vi "Begin.vi"() -> (0 "error out":errorcluster)   [LabVIEW 2013]
doc: "Called before other user functions, this VI is expected to open initial I/O refnums, load in file data, and do all program initialization. Notice that the <B>error out</B> terminal is simply used for data flow. Wiring it to other structures or subVIs ensures that this VI runs first."
uses:
  <vilib>/Rock Robotics/SystemInterfaces/DIO/FPGA_DIOPWMChannel.ctl
  <vilib>/Rock Robotics/WPI/DriverStation/WPI_DriverStationRobotMode2.ctl
  <vilib>/Rock Robotics/WPI/Joystick/WPI_JoystickDeviceEnum.ctl
  <vilib>/Rock Robotics/SystemInterfaces/DIO/FPGA_DIOChannel.ctl
  <vilib>/Rock Robotics/WPI/SafetyOutput/WPI_SafetyOutputConfigMenu.ctl
  <vilib>/Rock Robotics/SystemInterfaces/Typedef/FPGA_TypedefAnalogModule.ctl
  <vilib>/Rock Robotics/SystemInterfaces/AI/FPGA_AIChannel.ctl
  <vilib>/Rock Robotics/SystemInterfaces/Typedef/FPGA_TypedefAnalogModuleForGyro.ctl
  <vilib>/Rock Robotics/SystemInterfaces/AI/FPGA_AIGyroChannel.ctl
  <vilib>/Rock Robotics/SystemInterfaces/Typedef/FPGA_TypedefDigitalModule.ctl
  Robot Global Data.vi
  <vilib>/Rock Robotics/WPI/MotorControl/WPI_MotorControlOpen Jaguar.vi
  <vilib>/Rock Robotics/WPI/RobotDrive/WPI_RobotDriveOpen4MotorWithJaguar.vi
  <vilib>/Rock Robotics/WPI/MotorControl/WPI_MotorControlOpen Talon.vi
panel:
  out "error out 2":errorcluster
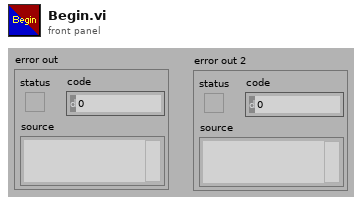
[diagram p1: front panel]
types:
  T1 = typedef "FPGA_DIOChannel.ctl" = enum8{"DIO 1", "DIO 2", "DIO 3", "DIO 4", "DIO 5", "DIO 6", "DIO 7", "DIO 8", "DIO 9", "DIO 10", "DIO 11", "DIO 12", "DIO 13", "DIO 14", "Invalid"}
  T2 = typedef "FPGA_TypedefDigitalModule.ctl" = enum16{"Digital Module 1", "Digital Module 2"}
  T3 = typedef "FPGA_AIGyroChannel.ctl" = enum8{"AI 1", "AI 2", "Invalid"}
  T4 = typedef "FPGA_TypedefAnalogModuleForGyro.ctl" = enum16{"Analog Module 1"}
  T5 = typedef "FPGA_AIChannel.ctl" = enum8{"AI 1", "AI 2", "AI 3", "AI 4", "AI 5", "AI 6", "AI 7", "AI 8", "Invalid"}
  T6 = typedef "FPGA_TypedefAnalogModule.ctl" = enum16{"Analog Module 1", "Analog Module 2"}
  T7 = typedef "WPI_SafetyOutputConfigMenu.ctl" = enum16{"Enable", "Disable"}
  T8 = typedef "FPGA_DIOPWMChannel.ctl" = enum8{"PWM 1", "PWM 2", "PWM 3", "PWM 4", "PWM 5", "PWM 6", "PWM 7", "PWM 8", "PWM 9", "PWM 10", "Invalid"}
  T9 = typedef "WPI_JoystickDeviceEnum.ctl" = enum16{"USB 1", "USB 2", "USB 3", "USB 4", "Kinect 1", "Kinect 2"}
  T10 = typedef "WPI_DriverStationRobotMode2.ctl" = enum16{"Autonomous Disabled", "Autonomous Enabled", "Teleop Disabled", "Teleop Enabled", "Timeout", "Finish", "Test Disabled", "Test Enabled"}
  T11 = typedef "WPI_GyroDevRef.ctl" = cluster{"DevStatus":errorcluster, "Analog Module":T6, "Analog Channel":T5, "Offset":dbl, "Gain (VoltsPerDegree/Second)":dbl}
  T12 = typedef "WPI_AnalogChannelDevRef.ctl" = cluster{"DevStatus":errorcluster, "Analog Module":T6, "Analog Channel":T5}
  T13 = typedef "WPI_RobotDriveDevRef.ctl" = cluster{"DevStatus":errorcluster, "Motors[]":T14[], "Square Inputs":bool, "Max Output":dbl, "Isochronous":bool}
  T14 = typedef "WPI_MotorControlDeviceRef.ctl" = cluster{"DeviceStatus":errorcluster, "Type":enum16{"PWM", "CAN"}, "PWM":cluster{"Digital Module":T2, "PWM Channel":T8, "DeadBand":T15}, "CAN":cluster{"Device Number":u8, "Control Mode":T16, "Semaphore":T17, "Max Vout":dbl}, "Invert":bool, "TransformRef":T18, "InvTransformRef":T18}
  T15 = typedef "WPI_PWMDeadband.ctl" = cluster{"Name":string, "maxPositivePwm":i32, "minPositivePwm":i32, "centerPwm":i32, "maxNegativePwm":i32, "minNegativePwm":i32, "angularRange":u16}
  T16 = typedef "WPI_CANJaguar_ControlMode.ctl" = enum8{"Percent VBus", "Current", "Speed", "Position", "Voltage"}
  T17 = typedef "Semaphore RefNum" = refnum<k1>
  T18 = typedef "WPI_PWMTransform_ConPane.ctl" = refnum<vi>
  T19 = typedef "WPI_JoystickDevRef.ctl" = cluster{"Device":T9}
  T20 = typedef "WPI_DigitalInputDevRef.ctl" = cluster{"DevStatus":errorcluster, "DIO Channel":T1, "Digital Module":T2}
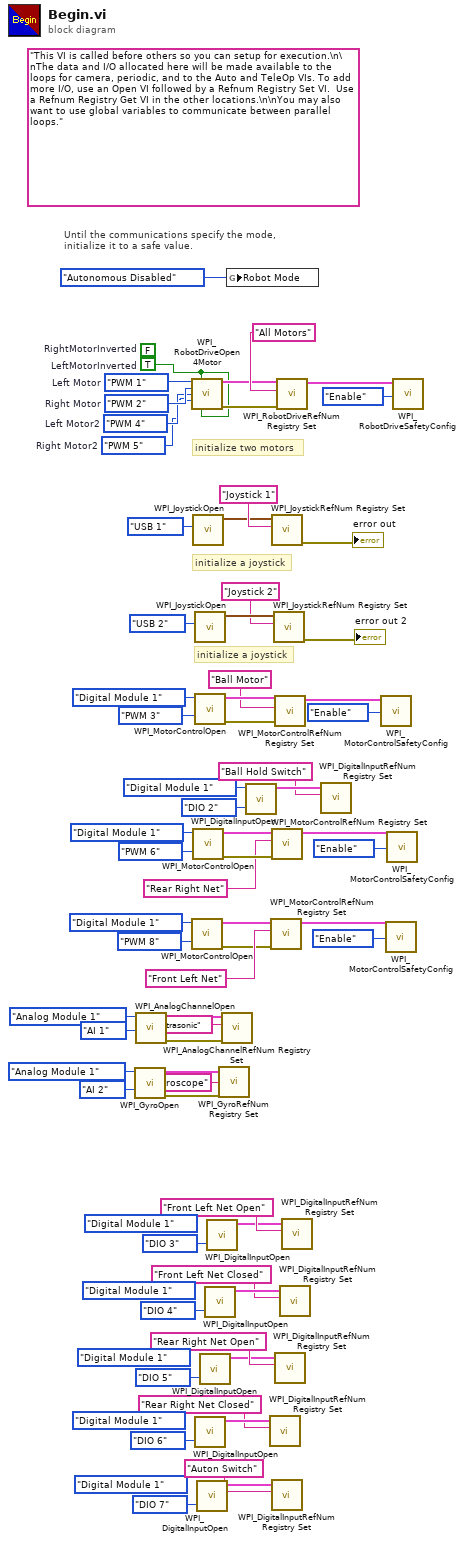
[diagram p0: block diagram]
diagram:
  (unwired) FPGA_TypedefDigitalModule."Digital Module 1" ("Digital Module (Module 1)")
  (unwired) FPGA_TypedefDigitalModule."Digital Module 1" ("Digital Module (Module 1)")
  (unwired) FPGA_TypedefDigitalModule."Digital Module 1" ("Digital Module (Module 1)")
  (unwired) FPGA_TypedefDigitalModule."Digital Module 1" ("Digital Module (Module 1)")
  (unwired) FPGA_TypedefDigitalModule."Digital Module 1" ("Digital Module (Module 1)")
  w43 = FPGA_DIOPWMChannel."PWM 5"  # Right Motor2
  w44 = FPGA_DIOPWMChannel."PWM 4"  # Left Motor2
  (unwired) "This VI is called before others so you can setup for execution.\n\nThe data and I/O allocated here will be made available to the loops for camera, periodic, and to the Auto and TeleOp VIs. To add more I/O, use an Open VI followed by a Refnum Registry Set VI.  Use a Refnum Registry Get VI in the other locations.\n\nYou may also want to use global variables to communicate between parallel loops."
  w45 = FPGA_DIOPWMChannel."PWM 2"  # Right Motor
  w46 = FPGA_DIOPWMChannel."PWM 1"  # Left Motor
  w40 = TRUE  # LeftMotorInverted
  (unwired) FALSE  # RightMotorInverted
  # "initialize a joystick"
  # "initialize a joystick"
  # "Until the communications specify the mode,\ninitialize it to a safe value."
  # "initialize two motors"
  n1 = call <vilib>:"WPI_GyroOpen.vi"("Analog Channel"=FPGA_AIGyroChannel."AI 2", "Analog Module (Module 1)"=FPGA_TypedefAnalogModuleForGyro."Analog Module 1") -> ("error out"=w17:errorcluster, "GyroDevRef"=w18:T11)  [unwired: 7 in, 1 out]
  n2 = call <vilib>:"WPI_AnalogChannelOpen.vi"("Analog Channel"=FPGA_AIChannel."AI 1", "Analog Module (Module 1)"=FPGA_TypedefAnalogModule."Analog Module 1") -> ("error out"=w21:errorcluster, "AIDeviceRef"=w23:T12)  [unwired: 8 in]
  n3 = call-poly <vilib>:"WPI_RobotDriveOpen4Motor.vi"("Rear Left Motor"=w46, "Rear Left Motor Inverted"=w40, "Rear Right Motor"=w45, "Front Left Motor"=w44, "Front Right Motor"=w43, "Front Left Motor Inverted"=w40) -> ("RobotDriveDevRef"=w42:T13, "error out"=w41:errorcluster)  [unwired: 8 in]
  n4 = call-poly <vilib>:"WPI_MotorControlOpen.vi"("PWM Channel"=FPGA_DIOPWMChannel."PWM 8", "Digital Module (Module 1)"=FPGA_TypedefDigitalModule."Digital Module 1") -> ("error out"=w28:errorcluster, "MotorControlDeviceRef"=w29:T14)  [unwired: 8 in]
  n5 = call <vilib>:"WPI_JoystickOpen.vi"("JoystickDevice"=WPI_JoystickDeviceEnum."USB 1") -> ("JoystickDevRef"=w64:T19)  [unwired: 10 in]
  n6 = call-poly <vilib>:"WPI_MotorControlOpen.vi"("PWM Channel"=FPGA_DIOPWMChannel."PWM 6", "Digital Module (Module 1)"=FPGA_TypedefDigitalModule."Digital Module 1") -> ("error out"=w37:errorcluster, "MotorControlDeviceRef"=w36:T14)  [unwired: 8 in]
  n7 = call <vilib>:"WPI_JoystickOpen.vi"("JoystickDevice"=WPI_JoystickDeviceEnum."USB 2") -> ("JoystickDevRef"=w59:T19)  [unwired: 10 in]
  n8 = call-poly <vilib>:"WPI_MotorControlOpen.vi"("PWM Channel"=FPGA_DIOPWMChannel."PWM 3", "Digital Module (Module 1)"=FPGA_TypedefDigitalModule."Digital Module 1") -> ("error out"=w55:errorcluster, "MotorControlDeviceRef"=w57:T14)  [unwired: 8 in]
  n9 = call <vilib>:"WPI_DigitalInputOpen.vi"("DIO Channel"=FPGA_DIOChannel."DIO 6") -> ("DigitalInputDevRef"=w5:T20)  [unwired: 9 in, 1 out]
  n10 = call <vilib>:"WPI_DigitalInputOpen.vi"("DIO Channel"=FPGA_DIOChannel."DIO 7") -> ("DigitalInputDevRef"=w2:T20)  [unwired: 9 in, 1 out]
  n11 = call <vilib>:"WPI_DigitalInputOpen.vi"("DIO Channel"=FPGA_DIOChannel."DIO 5") -> ("DigitalInputDevRef"=w8:T20)  [unwired: 9 in, 1 out]
  n12 = call <vilib>:"WPI_DigitalInputOpen.vi"("DIO Channel"=FPGA_DIOChannel."DIO 4") -> ("DigitalInputDevRef"=w11:T20)  [unwired: 9 in, 1 out]
  n13 = call <vilib>:"WPI_DigitalInputOpen.vi"("DIO Channel"=FPGA_DIOChannel."DIO 3") -> ("DigitalInputDevRef"=w14:T20)  [unwired: 9 in, 1 out]
  n14 = call <vilib>:"WPI_GyroRefNum Registry Set.vi"("error in (no error)"=w17, "refnum name"="Gyroscope", "GyroDevRef"=w18) -> ()  [unwired: 7 in, 2 out]
  n15 = call <vilib>:"WPI_AnalogChannelRefNum Registry Set.vi"("error in (no error)"=w21, "refnum name"="Ultrasonic", "AIDeviceRef"=w23) -> ()  [unwired: 7 in, 2 out]
  n16 = global write "Robot Global Data.vi" "Robot Mode"(WPI_DriverStationRobotMode2."Autonomous Disabled" ("Robot Mode")) -> ()
  n17 = call <vilib>:"WPI_DigitalInputOpen.vi"("DIO Channel"=FPGA_DIOChannel."DIO 2", "Digital Module (Module 1)"=FPGA_TypedefDigitalModule."Digital Module 1") -> ("DigitalInputDevRef"=w48:T20)  [unwired: 8 in, 1 out]
  n18 = call <vilib>:"WPI_DigitalInputRefNum Registry Set.vi"("refnum name"="Rear Right Net Closed", "DigitalInputDevRef"=w5) -> ()  [unwired: 8 in, 2 out]
  n19 = call <vilib>:"WPI_MotorControlRefNum Registry Set.vi"("error in (no error)"=w28, "refnum name"="Front Left Net", "MotorControlDevRef"=w29) -> ("MotorControlDevRef"=w32:T14)  [unwired: 7 in, 1 out]
  n20 = call <vilib>:"WPI_JoystickRefNum Registry Set.vi"("refnum name"="Joystick 1", "JoystickDevRef"=w64) -> ("error out"=→"error out":errorcluster)  [unwired: 8 in, 1 out]
  n21 = call <vilib>:"WPI_MotorControlRefNum Registry Set.vi"("error in (no error)"=w37, "refnum name"="Rear Right Net", "MotorControlDevRef"=w36) -> ("MotorControlDevRef"=w33:T14)  [unwired: 7 in, 1 out]
  n22 = call <vilib>:"WPI_DigitalInputRefNum Registry Set.vi"("refnum name"="Auton Switch", "DigitalInputDevRef"=w2) -> ()  [unwired: 8 in, 2 out]
  n23 = call <vilib>:"WPI_JoystickRefNum Registry Set.vi"("refnum name"="Joystick 2", "JoystickDevRef"=w59) -> ("error out"=→"error out 2":errorcluster)  [unwired: 8 in, 1 out]
  n24 = call <vilib>:"WPI_MotorControlRefNum Registry Set.vi"("error in (no error)"=w55, "refnum name"="Ball Motor", "MotorControlDevRef"=w57) -> ("MotorControlDevRef"=w52:T14)  [unwired: 7 in, 1 out]
  n25 = call <vilib>:"WPI_DigitalInputRefNum Registry Set.vi"("refnum name"="Rear Right Net Open", "DigitalInputDevRef"=w8) -> ()  [unwired: 8 in, 2 out]
  n26 = call <vilib>:"WPI_RobotDriveRefNum Registry Set.vi"("error in (no error)"=w41, "refnum name"="All Motors", "RobotDriveDevRef"=w42) -> ("RobotDriveDevRef"=w68:T13)  [unwired: 8 out]
  n27 = call <vilib>:"WPI_DigitalInputRefNum Registry Set.vi"("refnum name"="Front Left Net Closed", "DigitalInputDevRef"=w11) -> ()  [unwired: 8 in, 2 out]
  n28 = call <vilib>:"WPI_DigitalInputRefNum Registry Set.vi"("refnum name"="Front Left Net Open", "DigitalInputDevRef"=w14) -> ()  [unwired: 8 in, 2 out]
  n29 = call <vilib>:"WPI_DigitalInputRefNum Registry Set.vi"("refnum name"="Ball Hold Switch", "DigitalInputDevRef"=w48) -> ()  [unwired: 8 in, 2 out]
  n30 = call <vilib>:"WPI_MotorControlSafetyConfig.vi"("mode"=WPI_SafetyOutputConfigMenu."Enable", "MotorControlDevRef"=w52) -> ()  [unwired: 8 in, 2 out]
  n31 = call <vilib>:"WPI_MotorControlSafetyConfig.vi"("mode"=WPI_SafetyOutputConfigMenu."Enable", "MotorControlDevRef"=w32) -> ()  [unwired: 8 in, 2 out]
  n32 = call <vilib>:"WPI_MotorControlSafetyConfig.vi"("mode"=WPI_SafetyOutputConfigMenu."Enable", "MotorControlDevRef"=w33) -> ()  [unwired: 8 in, 2 out]
  n33 = call <vilib>:"WPI_RobotDriveSafetyConfig.vi"("mode"=WPI_SafetyOutputConfigMenu."Enable", "RobotDriveDevRef"=w68) -> ()  [unwired: 8 in, 2 out]
